vi "NicmosWriteMaskList.vi"(2 "Force Write Mask":bool, 9 "error in":errorcluster) -> (6 "error out":errorcluster)   [LabVIEW 2009]
doc: "Ce VI se charge d'écrire les masques spécifiées par Bank Window In si Bank Mask In est différent de la valeur par défaut dans NicmosMaskGlobal.vi\nCe VI utilise les références de VIs pour mettre à jour la valeur par défaut aprèe une ériture des masques sur la NICMOS."
uses:
  Controls/NICMOS.MASKBANKS.ctl
  NicmosGlobal.vi
  <vilib>/Utility/config.llb/NI_LVConfig.lvlib
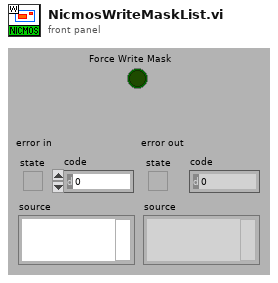
[diagram p1: front panel]
types:
  T1 = typedef "NICMOS.MASKBANKS.ctl" = cluster{"MaskList":cluster{"X":i32, "Y":i32, "NX":i32, "NY":i32}[], "Reform X":i32, "Reform Y":i32}[]
  T2 = typedef "NI_LVConfig.lvlib/Config Data RefNum.ctl" = refnum<k1>
  T3 = cluster{"Squares List":cluster{"X":i32, "Y":i32, "N":i32}[]}[]
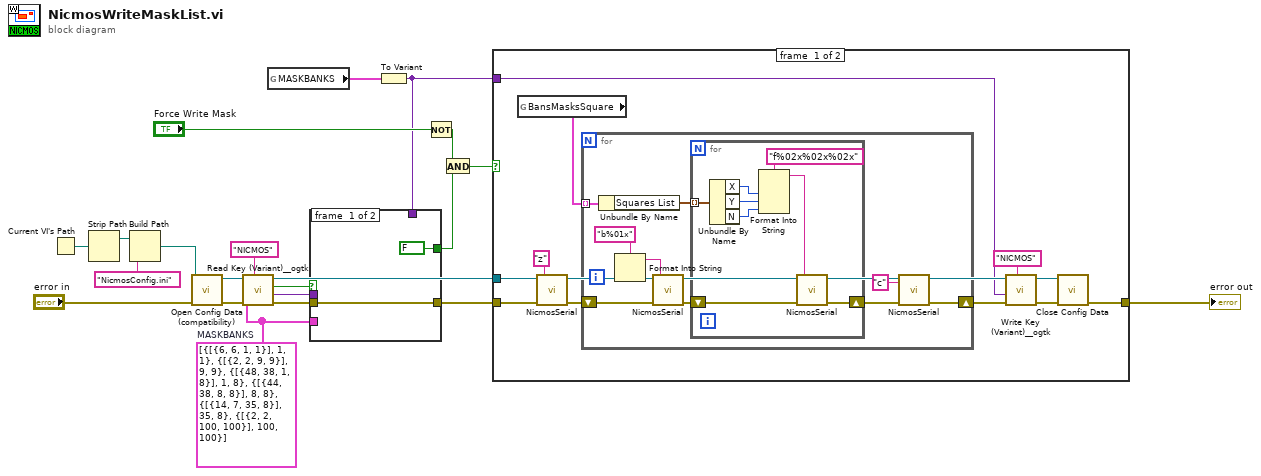
[diagram p0: block diagram]
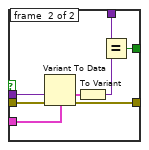
[diagram p2: hidden frame]
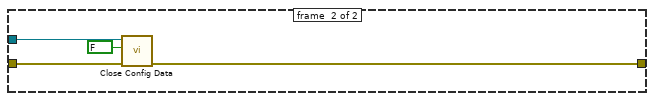
[diagram p3: hidden frame]
diagram:
  w2 = T1 [{"MaskList"=[{"X"=6, "Y"=6, "NX"=1, "NY"=1}], "Reform X"=1, "Reform Y"=1}, {"MaskList"=[{"X"=2, "Y"=2, "NX"=9, "NY"=9}], "Reform X"=9, "Reform Y"=9}, {"MaskList"=[{"X"=48, "Y"=38, "NX"=1, "NY"=8}], "Reform X"=1, "Reform Y"=8}, {"MaskList"=[{"X"=44, "Y"=38, "NX"=8, "NY"=8}], "Reform X"=8, "Reform Y"=8}, {"MaskList"=[{"X"=14, "Y"=7, "NX"=35, "NY"=8}], "Reform X"=35, "Reform Y"=8}, {"MaskList"=[{"X"=2, "Y"=2, "NX"=100, "NY"=100}], "Reform X"=100, "Reform Y"=100}]  # MASKBANKS
  n1 = Current VI's Path() -> (path=w17:path)
  n2 = Strip Path(path=w17) -> (stripped path=w15:path)  [unwired: 1 out]
  n3 = Build Path(base path=w15, name or relative path="NicmosConfig.ini" ("nom ou chemin relatif")) -> (appended path=w14:path)
  n4 = call <vilib>:"Open Config Data (compatibility).vi"("error in (no error)"="error in", "configuration file path"=w14) -> ("error out"=w13:errorcluster, "refnum"=w12:T2)  [unwired: 7 in, 1 out]
  n5 = call <userlib>:"Read Key (Variant)__ogtk.vi"("section"="NICMOS", "error in (no error)"=w13, "type"=w2, "refnum"=w12) -> ("error out"=w5:errorcluster, "key-value"=w3:variant, "found?"=w1:bool, "refnum out"=w10:T2)  [unwired: 4 in]
  n6 = global read "NicmosGlobal.vi" "MASKBANKS"() -> (w8:T1)
  n7 = To Variant(anything=w8) -> (Variant=w7:variant)
  n8 = case shown="False" w1 {
    tunnel: [FALSE w31] -> w9
    tunnel: w7 -> [_ w30]
    tunnel: w5 -> [w23 w29]
    tunnel: [w23 w28] -> w4
    tunnel: w3 -> [_ w27]
    tunnel: w2 -> [_ w24]
    frame #0 {
    }
    frame #1 {
      n9 = Variant To Data(error in=w29, Variant=w27, type=w24) -> (error out=w28:errorcluster, data=w26:T1)
      n10 = To Variant(anything=w26) -> (Variant=w25:variant)
      n11 = Equal?(x=w30, y=w25) -> (x = y?=w31:bool)
    }
  }
  n12 = Not(x="Force Write Mask") -> (.not. x?=w20:bool)
  n13 = And(x=w20, y=w9) -> (x .and. y?=w19:bool)
  n14 = case shown="False" w19 {
    tunnel: w4 -> [w42 w63]
    tunnel: [w32 w62] -> w6
    tunnel: w10 -> [w37 w64]
    tunnel: w7 -> [w36 _]
    frame #0 {
      n15 = global read "NicmosGlobal.vi" "BansMasksSquare"() -> (w39:T3)
      n16 = call "NicmosSerial.vi"("error in"=w42, "Command"="z") -> ("error out"=w40:errorcluster)  [unwired: 3 in, 1 out]
      n17 = for {
        shift-right: [w44] -> w38
        shift-left: w40 -> [w50]
        tunnel: w39 -> [w52] mode=indexing
        i -> [w47]
        n18 = Unbundle By Name(w52) -> ("Squares List"=w51:cluster{"X":i32, "Y":i32, "N":i32}[])
        n19 = Format Into String(format string="b%01x" ("Chaîne d'entrée"), w47) -> (resulting string=w48:string)  [unwired: 2 in, 1 out]
        n20 = call "NicmosSerial.vi"("error in"=w50, "Command"=w48) -> ("error out"=w49:errorcluster)  [unwired: 3 in, 1 out]
        n21 = for {
          shift-right: [w57] -> w45
          shift-left: w49 -> [w58]
          tunnel: w51 -> [w56] mode=indexing
          n22 = Unbundle By Name(w56) -> ("X"=w54:i32, "Y"=w55:i32, "N"=w53:i32)
          n23 = Format Into String(format string="f%02x%02x%02x" ("Question F"), w54, w55, w53) -> (resulting string=w60:string)  [unwired: 2 in, 1 out]
          n24 = call "NicmosSerial.vi"("error in"=w58, "Command"=w60) -> ("error out"=w57:errorcluster)  [unwired: 3 in, 1 out]
        }
        n25 = call "NicmosSerial.vi"("error in"=w45, "Command"="c") -> ("error out"=w44:errorcluster)  [unwired: 3 in, 1 out]
      }
      n26 = call <userlib>:"Write Key (Variant)__ogtk.vi"("section"="NICMOS", "error in (no error)"=w38, "key-value"=w36, "refnum"=w37) -> ("error out"=w33:errorcluster, "refnum out"=w34:T2)  [unwired: 6 in]
      n27 = call <vilib>:"Close Config Data.vi"("error in (no error)"=w33, "refnum"=w34) -> ("error out"=w32:errorcluster)  [unwired: 8 in, 1 out]
    }
    frame #1 {
      n28 = call <vilib>:"Close Config Data.vi"("error in (no error)"=w63, "write file if changed (T)"=FALSE ("write configuration file? (T)"), "refnum"=w64) -> ("error out"=w62:errorcluster)  [unwired: 7 in, 1 out]
    }
  }
  "error out" <- w6
